vi "Edge Distance.vi"(7 "error in (no error)":errorcluster, 8 "Cluster":T7={"Center X &Y"={"Center X"=0.0, "Center Y"=0.0}, "ROI Ref [Before Transformation]"={"Global Rectangle"=[], "Contours"=[]}, "Edge Options ROI Ref"={"Edge Polarity"=2, "Kernel Size"=3, "Width"=3, "Minimum Edge Strength"=30.0, "Interpolation Type"=enum."Zero Order", "Data Processing Method"=enum."Average"}, "Line Options ROI Ref"={"Number of Lines"=1, "Type"=enum."Best Edge Rake", "Min. Score"=10.0, "Max. Score"=1000.0, "Orientation"=0.0, "Angle Range"=10.0, "Angle Tolerance"=1.0, "Step Size"=3, "Min. SNR (db)"=0.0, "Min. Points (%)"=25.0, "Hough Iterations"=5}, "Search Direction ROI Ref"=2, "Meas ROI 1[Before Transformation]"={"Global Rectangle"=[], "Contours"=[]}, "Edge Options ROI 1"={"Edge Polarity"=2, "Kernel Size"=3, "Width"=3, "Minimum Edge Strength"=30.0, "Interpolation Type"=enum."Zero Order", "Data Processing Method"=enum."Average"}, "Line Options ROI 1"={"Number of Lines"=1, "Type"=enum."Best Edge Rake", "Min. Score"=10.0, "Max. Score"=1000.0, "Orientation"=0.0, "Angle Range"=10.0, "Angle Tolerance"=1.0, "Step Size"=3, "Min. SNR (db)"=0.0, "Min. Points (%)"=25.0, "Hough Iterations"=5}, "Search Direction ROI 1"=2, "Meas ROI 2[Before Transformation]"={"Global Rectangle"=[], "Contours"=[]}, "Edge Options ROI 2"={"Edge Polarity"=2, "Kernel Size"=3, "Width"=3, "Minimum Edge Strength"=30.0, "Interpolation Type"=enum."Zero Order", "Data Processing Method"=enum."Average"}, "Line Options ROI 2"={"Number of Lines"=1, "Type"=enum."Best Edge Rake", "Min. Score"=10.0, "Max. Score"=1000.0, "Orientation"=0.0, "Angle Range"=10.0, "Angle Tolerance"=1.0, "Step Size"=3, "Min. SNR (db)"=0.0, "Min. Points (%)"=25.0, "Hough Iterations"=5}, "Search Direction ROI 2"=2} {"ROI Ref [Before Transformation]"."Contours"."Type" items=["No Selection", "Point", "Line", "Rectangle", "Oval", "Polygon", "Freehand Region", "Annulus", "Unused2", "Unused3", "Broken Line", "Freehand Line", "Rotated Rectangle"]; "Edge Options ROI Ref"."Edge Polarity" items=["All Edges", "Rising Edges", "Falling Edges"]; "Edge Options ROI Ref"."Minimum Edge Strength" format="%.2f"; "Edge Options ROI Ref"."Width" step=2; "Edge Options ROI Ref"."Kernel Size" step=2; "Line Options ROI Ref"."Min. Points (%)" min=0.0 max=100.0; "Line Options ROI Ref"."Min. SNR (db)" min=0.0; "Line Options ROI Ref"."Max. Score" min=0.0 max=1024.0; "Line Options ROI Ref"."Min. Score" min=0.0 max=1024.0 step=1.0; "Search Direction ROI Ref" items=["Left to Right", "Right to Left", "Top to Bottom", "Bottom to Top"]; "Meas ROI 1[Before Transformation]"."Contours"."Type" items=["No Selection", "Point", "Line", "Rectangle", "Oval", "Polygon", "Freehand Region", "Annulus", "Unused2", "Unused3", "Broken Line", "Freehand Line", "Rotated Rectangle"]; "Edge Options ROI 1"."Edge Polarity" items=["All Edges", "Rising Edges", "Falling Edges"]; "Edge Options ROI 1"."Minimum Edge Strength" format="%.2f"; "Edge Options ROI 1"."Width" step=2; "Edge Options ROI 1"."Kernel Size" step=2; "Line Options ROI 1"."Min. Points (%)" min=0.0 max=100.0; "Line Options ROI 1"."Min. SNR (db)" min=0.0; "Line Options ROI 1"."Max. Score" min=0.0 max=1024.0; "Line Options ROI 1"."Min. Score" min=0.0 max=1024.0 step=1.0; "Search Direction ROI 1" items=["Left to Right", "Right to Left", "Top to Bottom", "Bottom to Top"]; "Meas ROI 2[Before Transformation]"."Contours"."Type" items=["No Selection", "Point", "Line", "Rectangle", "Oval", "Polygon", "Freehand Region", "Annulus", "Unused2", "Unused3", "Broken Line", "Freehand Line", "Rotated Rectangle"]; "Edge Options ROI 2"."Edge Polarity" items=["All Edges", "Rising Edges", "Falling Edges"]; "Edge Options ROI 2"."Minimum Edge Strength" format="%.2f"; "Edge Options ROI 2"."Width" step=2; "Edge Options ROI 2"."Kernel Size" step=2; "Line Options ROI 2"."Min. Points (%)" min=0.0 max=100.0; "Line Options ROI 2"."Min. SNR (db)" min=0.0; "Line Options ROI 2"."Max. Score" min=0.0 max=1024.0; "Line Options ROI 2"."Min. Score" min=0.0 max=1024.0 step=1.0; "Search Direction ROI 2" items=["Left to Right", "Right to Left", "Top to Bottom", "Bottom to Top"]}, 9 "Calibration Image":T1(plugin-control), 10 "Input Image":T1(plugin-control)) -> (0 "error out":errorcluster, 2 "Input Image 2":T1(plugin-control), 3 "output cluster":T8)   [LabVIEW 2019, in "Algorithm.lvclass"]
uses:
  FrameworkOverrides/Algorithm.lvclass
  <vilib>/vision/NI_Vision_Development_Module.lvlib
  <vilib>/vision/Measure.llb/Straight Edge Process.ctl
  <vilib>/vision/Measure.llb/Straight Edge Options.ctl
  <vilib>/vision/Measure.llb/Edge Polarity.ctl
  <vilib>/vision/Measure.llb/Edge Options.ctl
  <vilib>/vision/Image Controls.llb/IMAQ Image.ctl
panel:
  out "Image (duplicate)":T1
  out "Angle (Pixel)":dbl
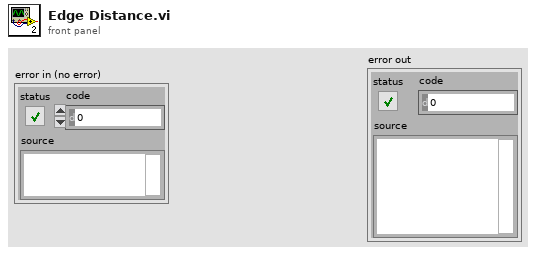
[diagram p1: front panel]
types:
  T1 = typedef "IMAQ Image.ctl" = refnum<image>
  T2 = typedef "ROI Descriptor" = cluster{"Global Rectangle":i32[], "Contours":cluster{"ID":enum32{"External", "Internal"}, "Type":u32, "Coordinates":i32[]}[]}
  T3 = typedef "Edge Options.ctl" = cluster{"Edge Polarity":T4, "Kernel Size":u32, "Width":u32, "Minimum Edge Strength":sgl, "Interpolation Type":enum32{"Zero Order", "Bilinear", "Quadratic", "Cubic", "Bilinear Fixed"}, "Data Processing Method":enum32{"Average", "Median"}}
  T4 = typedef "Edge Polarity.ctl" = u32
  T5 = typedef "Straight Edge Options.ctl" = cluster{"Number of Lines":i32, "Type":T6, "Min. Score":dbl, "Max. Score":dbl, "Orientation":dbl, "Angle Range":dbl, "Angle Tolerance":dbl, "Step Size":u32, "Min. SNR (db)":dbl, "Min. Points (%)":dbl, "Hough Iterations":i32}
  T6 = typedef "Straight Edge Process.ctl" = enum32{"First Edge Rake", "Best Edge Rake", "Hough Edge Rake", "First Edge Projection", "Best Edge Projection"}
  T7 = cluster{"Center X &Y":cluster{"Center X":dbl, "Center Y":dbl}, "ROI Ref [Before Transformation]":T2, "Edge Options ROI Ref":T3, "Line Options ROI Ref":T5, "Search Direction ROI Ref":u32, "Meas ROI 1[Before Transformation]":T2, "Edge Options ROI 1":T3, "Line Options ROI 1":T5, "Search Direction ROI 1":u32, "Meas ROI 2[Before Transformation]":T2, "Edge Options ROI 2":T3, "Line Options ROI 2":T5, "Search Direction ROI 2":u32}
  T8 = cluster{"Points for Overlay":cluster{"Point 2":cluster{"X":sgl, "Y":sgl}, "Point 2":cluster{"X":sgl, "Y":sgl}}, "Measurement":sgl}
  T9 = cluster{"Left":dbl, "Top":dbl, "Right":dbl, "Bottom":dbl, "Angle":dbl}
  T10 = cluster{"Point 1":cluster{"X":sgl, "Y":sgl}, "Point 2":cluster{"X":sgl, "Y":sgl}}
  T11 = cluster{"ID":enum32{"External", "Internal"}, "Type":u32, "Coordinates":i32[]}[]
  T12 = cluster{"ID":enum32{"External", "Internal"}, "Type":u32, "Coordinates":i32[]}
  T13 = cluster{"Coordinates[0]":i32, "Coordinates[1]":i32, "Coordinates[2]":i32, "Coordinates[3]":i32, "Coordinates[4]":i32}
  T14 = cluster{"Point1 (Pixels)":cluster{"X":sgl, "Y":sgl}, "Point2 (Pixels)":cluster{"X":sgl, "Y":sgl}, "Point1 (Real-World)":cluster{"X":sgl, "Y":sgl}, "Point2 (Real-World)":cluster{"X":sgl, "Y":sgl}, "Angle (Pixel)":dbl, "Angle (Real-World)":dbl, "Score":dbl, "Straightness":dbl, "Average SNR (db)":dbl, "Calibration Valid":bool}[]
  T15 = cluster{"Point1 (Pixels)":cluster{"X":sgl, "Y":sgl}, "Point2 (Pixels)":cluster{"X":sgl, "Y":sgl}, "Point1 (Real-World)":cluster{"X":sgl, "Y":sgl}, "Point2 (Real-World)":cluster{"X":sgl, "Y":sgl}, "Angle (Pixel)":dbl, "Angle (Real-World)":dbl, "Score":dbl, "Straightness":dbl, "Average SNR (db)":dbl, "Calibration Valid":bool}
  T16 = cluster{"Point 2":cluster{"X":sgl, "Y":sgl}, "Point 2":cluster{"X":sgl, "Y":sgl}}
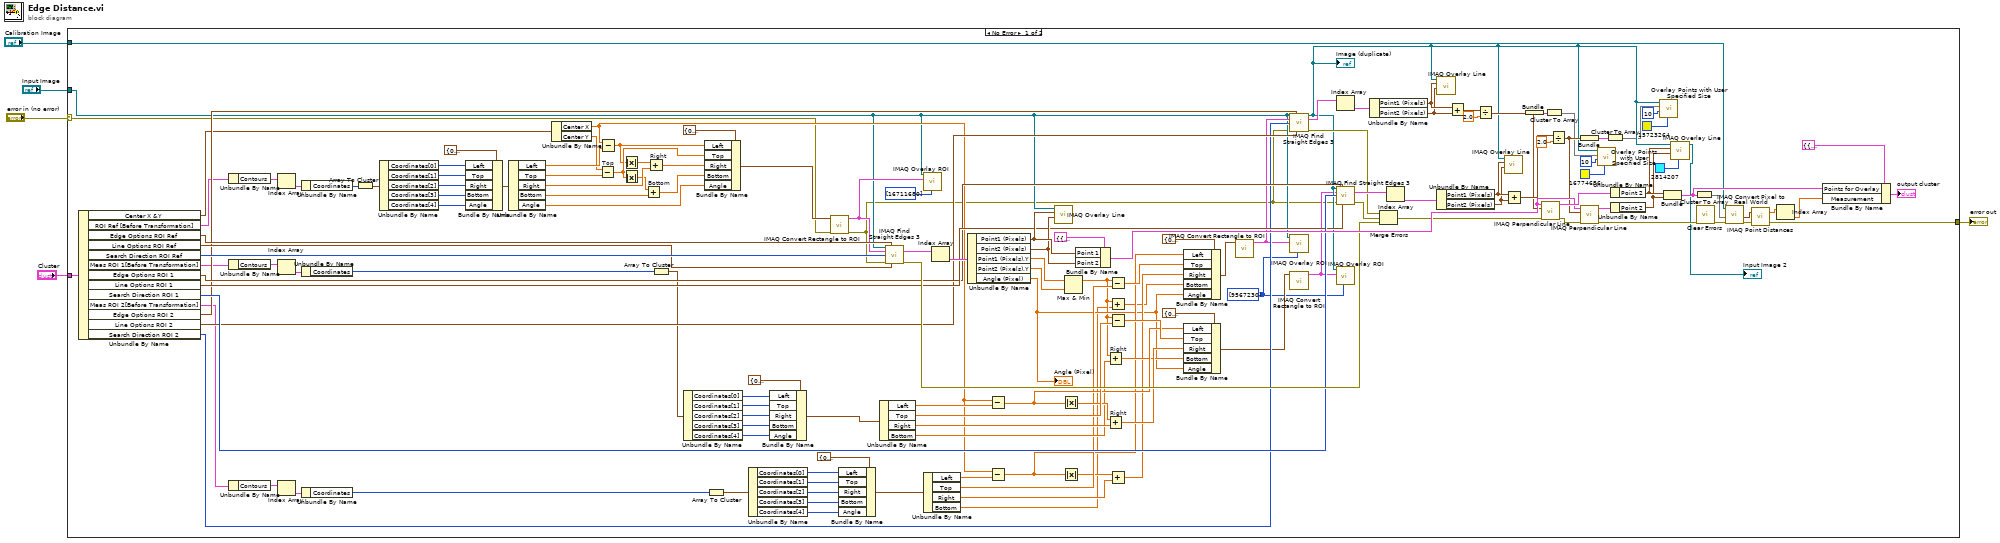
[diagram p0: block diagram]
diagram:
  n1 = case shown="No Error" "error in (no error)" {
    selector: "error in (no error)" -> [w21 w154]
    tunnel: [w130 w154] -> w5
    tunnel: "Input Image" -> [w15 _]
    tunnel: "Calibration Image" -> [w121 _]
    tunnel: "Cluster" -> [w109 _]
    frame No Error {
      w18 = u32[] [9567230] ("Colors (Green)")
      n2 = Unbundle By Name(w109) -> ("Center X &Y"=w65:cluster{"Center X":dbl, "Center Y":dbl}, "ROI Ref [Before Transformation]"=w98:T2, "Edge Options ROI Ref"=w107:T3, "Line Options ROI Ref"=w106:T5, "Search Direction ROI Ref"=w108:u32, "Meas ROI 1[Before Transformation]"=w93:T2, "Edge Options ROI 1"=w103:T3, "Line Options ROI 1"=w104:T5, "Search Direction ROI 1"=w105:u32, "Meas ROI 2[Before Transformation]"=w99:T2, "Edge Options ROI 2"=w102:T3, "Line Options ROI 2"=w101:T5, "Search Direction ROI 2"=w100:u32)
      n3 = Unbundle By Name(w98) -> ("Contours"=w97:T11)
      n4 = Unbundle By Name(w93) -> ("Contours"=w92:T11)
      n5 = Unbundle By Name(w99) -> ("Contours"=w88:T11)
      n6 = Index Array(array=w97) -> (element=w96:T12)  [unwired: 1 in]
      n7 = Index Array(array=w92) -> (element=w91:T12)  [unwired: 1 in]
      n8 = Index Array(array=w88) -> (element=w87:T12)  [unwired: 1 in]
      n9 = Unbundle By Name(w96) -> ("Coordinates"=w95:i32[])
      n10 = Unbundle By Name(w91) -> ("Coordinates"=w90:i32[])
      n11 = Unbundle By Name(w87) -> ("Coordinates"=w86:i32[])
      n12 = Array To Cluster(array=w95) -> (cluster=w94:T13)
      n13 = Unbundle By Name(w94) -> ("Coordinates[0]"=w83:i32, "Coordinates[1]"=w82:i32, "Coordinates[2]"=w81:i32, "Coordinates[3]"=w80:i32, "Coordinates[4]"=w79:i32)
      n14 = Bundle By Name(cluster=T9 {"Left"=0.0, "Top"=0.0, "Right"=0.0, "Bottom"=0.0, "Angle"=0.0} ("input cluster"), "Left"=w83, "Top"=w82, "Right"=w81, "Bottom"=w80, "Angle"=w79) -> (w66:T9)
      n15 = Unbundle By Name "Unbundle By Name"(w66) -> ("Left"=w74:dbl, "Top"=w75:dbl, "Right"=w76:dbl, "Bottom"=w77:dbl, "Angle"=w78:dbl)
      n16 = Unbundle By Name(w65) -> ("Center X"=w34:dbl, "Center Y"=w64:dbl)
      n17 = Subtract "Top"(x=w64, y=w75) -> (x-y=w71:dbl)
      n18 = Subtract(x=w34, y=w74) -> (x-y=w70:dbl)
      n19 = Absolute Value(x=w70) -> (abs(x)=w67:dbl)
      n20 = Absolute Value(x=w71) -> (abs(x)=w68:dbl)
      n21 = Add "Bottom"(x=w68, y=w77) -> (x+y=w73:dbl)
      n22 = Add "Right"(x=w67, y=w76) -> (x+y=w72:dbl)
      n23 = Array To Cluster(array=w90) -> (cluster=w89:T13)
      n24 = Unbundle By Name(w89) -> ("Coordinates[0]"=w54:i32, "Coordinates[1]"=w55:i32, "Coordinates[2]"=w56:i32, "Coordinates[3]"=w57:i32, "Coordinates[4]"=w59:i32)
      n25 = Bundle By Name(cluster=T9 {"Left"=0.0, "Top"=0.0, "Right"=0.0, "Bottom"=0.0, "Angle"=0.0} ("input cluster"), "Left"=w70, "Top"=w71, "Right"=w72, "Bottom"=w73, "Angle"=w78) -> (w63:T9)
      n26 = Array To Cluster(array=w86) -> (cluster=w85:T13)
      n27 = Unbundle By Name(w85) -> ("Coordinates[0]"=w41:i32, "Coordinates[1]"=w40:i32, "Coordinates[2]"=w39:i32, "Coordinates[3]"=w38:i32, "Coordinates[4]"=w37:i32)
      n28 = Bundle By Name(cluster=T9 {"Left"=0.0, "Top"=0.0, "Right"=0.0, "Bottom"=0.0, "Angle"=0.0} ("input cluster"), "Left"=w54, "Top"=w55, "Right"=w56, "Bottom"=w57, "Angle"=w59) -> (w58:T9)
      n29 = call "IMAQ Convert Rectangle to ROI"("error in (no error)"=w21, "Rectangle"=w63) -> ("error out"=w13:errorcluster, "ROI Descriptor"=w16:T2)  [unwired: 7 in]
      n30 = Bundle By Name(cluster=T9 {"Left"=0.0, "Top"=0.0, "Right"=0.0, "Bottom"=0.0, "Angle"=0.0} ("input cluster"), "Left"=w41, "Top"=w40, "Right"=w39, "Bottom"=w38, "Angle"=w37) -> (w36:T9)
      n31 = Unbundle By Name "Unbundle By Name"(w58) -> ("Left"=w51:dbl, "Top"=w50:dbl, "Right"=w46:dbl, "Bottom"=w44:dbl)
      n32 = call "IMAQ Find Straight Edges 3"("Image"=w15, "Edge Options"=w107, "ROI Descriptor"=w16, "Search Direction"=w108, "error in (no error)"=w13, "Line Options"=w106) -> ("Straight Edges"=w125:T14, "error out"=w122:errorcluster)  [unwired: 5 in, 3 out]
      n33 = call "IMAQ Overlay ROI"("Colors (Green)"=u32[] [16711680], "ROI Descriptor"=w16, "Image"=w15) -> ()  [unwired: 7 in, 2 out]
      n34 = Unbundle By Name(w36) -> ("Left"=w33:dbl, "Top"=w32:dbl, "Right"=w28:dbl, "Bottom"=w24:dbl)
      n35 = Index Array(array=w125) -> (element=w145:T15)  [unwired: 1 in]
      n36 = Unbundle By Name(w145) -> ("Point1 (Pixels)"=w124:cluster{"X":sgl, "Y":sgl}, "Point2 (Pixels)"=w123:cluster{"X":sgl, "Y":sgl}, "Point1 (Pixels).Y"=w62:sgl, "Point2 (Pixels).Y"=w61:sgl, "Angle (Pixel)"=w26:dbl)
      "Angle (Pixel)" <- w26
      n37 = Subtract(x=w34, y=w51) -> (x-y=w48:dbl)
      n38 = Subtract(x=w34, y=w33) -> (x-y=w30:dbl)
      n39 = call "IMAQ Overlay Line"("End Point"=w123, "Start Point"=w124, "Image"=w15) -> ()  [unwired: 7 in, 2 out]
      n40 = Absolute Value(x=w48) -> (abs(x)=w47:dbl)
      n41 = Absolute Value(x=w30) -> (abs(x)=w29:dbl)
      n42 = Max & Min(x=w62, y=w61) -> (max(x,y)=w25:sgl)  [unwired: 1 out]
      n43 = Bundle By Name(cluster=T10 {"Point 1"={"X"=0.0, "Y"=0.0}, "Point 2"={"X"=0.0, "Y"=0.0}} ("Line"), "Point 1"=w124, "Point 2"=w123) -> (w151:T10)
      n44 = Add "Right"(x=w25, y=w44) -> (x+y=w43:dbl)
      n45 = Add "Right"(x=w47, y=w46) -> (x+y=w45:dbl)
      n46 = Subtract(x=w25, y=w32) -> (x-y=w31:dbl)
      n47 = Add(x=w25, y=w24) -> (x+y=w23:dbl)
      n48 = Subtract(x=w25, y=w50) -> (x-y=w49:dbl)
      n49 = Add(x=w29, y=w28) -> (x+y=w27:dbl)
      n50 = Bundle By Name(cluster=T9 {"Left"=0.0, "Top"=0.0, "Right"=0.0, "Bottom"=0.0, "Angle"=0.0} ("input cluster"), "Left"=w30, "Top"=w31, "Right"=w27, "Bottom"=w23, "Angle"=w26) -> (w22:T9)
      n51 = Bundle By Name(cluster=T9 {"Left"=0.0, "Top"=0.0, "Right"=0.0, "Bottom"=0.0, "Angle"=0.0} ("input cluster"), "Left"=w48, "Top"=w49, "Right"=w45, "Bottom"=w43, "Angle"=w26) -> (w52:T9)
      n52 = call "IMAQ Convert Rectangle to ROI"("Rectangle"=w22) -> ("ROI Descriptor"=w17:T2)  [unwired: 8 in, 1 out]
      n53 = call "IMAQ Find Straight Edges 3"("Image"=w15, "Edge Options"=w102, "ROI Descriptor"=w17, "Search Direction"=w100, "error in (no error)"=w13, "Line Options"=w101) -> ("Image (duplicate)"=w20:T1, "Straight Edges"=w141:T14, "error out"=w140:errorcluster)  [unwired: 5 in, 2 out]
      "Image (duplicate)" <- w20
      n54 = call "IMAQ Overlay ROI"("Colors (Green)"=w18, "ROI Descriptor"=w17, "Image"=w15) -> ()  [unwired: 7 in, 2 out]
      n55 = call "IMAQ Convert Rectangle to ROI"("Rectangle"=w52) -> ("ROI Descriptor"=w19:T2)  [unwired: 8 in, 1 out]
      n56 = Index Array(array=w141) -> (element=w142:T15)  [unwired: 1 in]
      n57 = call "IMAQ Find Straight Edges 3"("Image"=w20, "Edge Options"=w103, "ROI Descriptor"=w19, "Search Direction"=w105, "error in (no error)"=w13, "Line Options"=w104) -> ("Straight Edges"=w144:T14, "error out"=w139:errorcluster)  [unwired: 5 in, 3 out]
      n58 = call "IMAQ Overlay ROI"("Colors (Green)"=w18, "ROI Descriptor"=w19, "Image"=w20) -> ()  [unwired: 7 in, 2 out]
      n59 = Unbundle By Name(w142) -> ("Point1 (Pixels)"=w129:cluster{"X":sgl, "Y":sgl}, "Point2 (Pixels)"=w128:cluster{"X":sgl, "Y":sgl})
      n60 = Merge Errors(w140, w139, w122) -> (w10:errorcluster)
      n61 = Index Array(array=w144) -> (element=w143:T15)  [unwired: 1 in]
      n62 = call "IMAQ Overlay Line"("End Point"=w128, "Start Point"=w129, "Image"=w20) -> ()  [unwired: 7 in, 2 out]
      n63 = Unbundle By Name(w143) -> ("Point1 (Pixels)"=w127:cluster{"X":sgl, "Y":sgl}, "Point2 (Pixels)"=w126:cluster{"X":sgl, "Y":sgl})
      n64 = Add(x=w129, y=w128) -> (x+y=w147:cluster{"X":sgl, "Y":sgl})
      n65 = Divide(x=w147, y=2.0) -> (x/y=w117:cluster{"X":dbl, "Y":dbl})
      n66 = call "IMAQ Overlay Line"("End Point"=w126, "Start Point"=w127, "Image"=w20) -> ()  [unwired: 7 in, 2 out]
      n67 = Add(x=w127, y=w126) -> (x+y=w148:cluster{"X":sgl, "Y":sgl})
      n68 = Bundle(w117) -> (w116:cluster{cluster{"X":dbl, "Y":dbl}})  [unwired: 1 in]
      n69 = call "IMAQ Perpendicular Line"("error in (no error)"=w10, "Point"=w117, "Line"=w151) -> ("error out"=w9:errorcluster, "Perpendicular Line"=w152:T10)  [unwired: 6 in, 1 out]
      n70 = Cluster To Array(cluster=w116) -> (array=w7:cluster{"X":dbl, "Y":dbl}[])
      n71 = Divide(x=w148, y=2.0) -> (x/y=w115:cluster{"X":dbl, "Y":dbl})
      n72 = Bundle(w115) -> (w114:cluster{cluster{"X":dbl, "Y":dbl}})  [unwired: 1 in]
      n73 = call "IMAQ Perpendicular Line"("error in (no error)"=w9, "Point"=w115, "Line"=w151) -> ("error out"=w12:errorcluster, "Perpendicular Line"=w153:T10)  [unwired: 6 in, 1 out]
      n74 = call "Overlay Points with User Specified Size.vi"("Color"=u32 16774656, "Point Diameter (5)"=u32 10, "Points"=w7, "Image In"=w20) -> ()  [unwired: 6 in, 2 out]
      n75 = Cluster To Array(cluster=w114) -> (array=w6:cluster{"X":dbl, "Y":dbl}[])
      n76 = Unbundle By Name(w152) -> ("Point 2"=w120:cluster{"X":sgl, "Y":sgl})
      n77 = Unbundle By Name(w153) -> ("Point 2"=w119:cluster{"X":sgl, "Y":sgl})
      n78 = call "Overlay Points with User Specified Size.vi"("Color"=u32 15723264, "Point Diameter (5)"=u32 10, "Points"=w6, "Image In"=w20) -> ()  [unwired: 6 in, 2 out]
      n79 = Bundle("Point 2"=w120, "Point 2"=w119) -> (w132:T16)  [unwired: 1 in]
      n80 = call "IMAQ Overlay Line"("Color"=u32 2814207, "End Point"=w119, "Start Point"=w120, "Image"=w20) -> ("Image Out"=→"Input Image 2":T1)  [unwired: 6 in, 1 out]
      n81 = Cluster To Array(cluster=w132) -> (array=w133:cluster{"X":sgl, "Y":sgl}[])
      n82 = call <vilib>:"Clear Errors.vi"("error in (no error)"=w12) -> ("error out"=w11:errorcluster)  [unwired: 5 in, 1 out]
      n83 = call "IMAQ Convert Pixel to Real World"("error in (no error)"=w11, "Array of Pixel Coordinates"=w133, "Calibrated Image"=w121) -> ("error out"=w137:errorcluster, "Array of Real World Coordinates"=w138:cluster{"X":sgl, "Y":sgl}[])  [unwired: 3 in, 4 out]
      n84 = call "IMAQ Point Distances"("Points"=w138, "error in (no error)"=w137) -> ("Distances"=w136:sgl[], "error out"=w130:errorcluster)  [unwired: 3 in]
      n85 = Index Array(array=w136) -> (element=w134:sgl)  [unwired: 1 in]
      n86 = Bundle By Name(cluster=T8 {"Points for Overlay"={"Point 2"={"X"=0.0, "Y"=0.0}, "Point 2"={"X"=0.0, "Y"=0.0}}, "Measurement"=0.0}, "Points for Overlay"=w132, "Measurement"=w134) -> (→"output cluster":T8)
    }
    frame Error {
    }
  }
  "error out" <- w5
